vi "ResistanceEquivalent.vi"(3 "Connect":enum16{"SZEREGOWO", "RÓWNOLEGLE"}(ring) caption="Rodzaj po³¹czenia", 4 "R":dbl[](array[numeric]) caption="R [Ohm]") -> (0 "R_eq":dbl caption="R_Z [Ohm]" format="%#.2g")   [LabVIEW 2020]
doc: "Ten subVI liczy opór zastepczy."
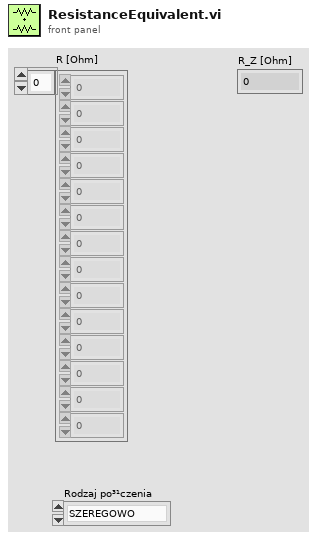
[diagram p1: front panel]
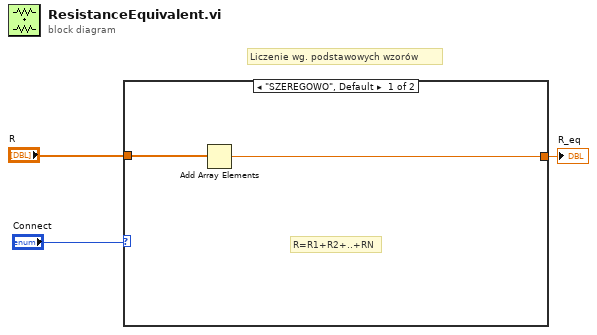
[diagram p0: block diagram]
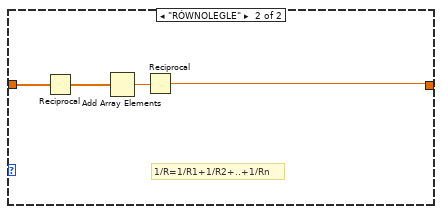
[diagram p2: hidden frame]
diagram:
  # "Liczenie wg. podstawowych wzorów"
  n1 = case shown="\"SZEREGOWO\", Default" "Connect" {
    tunnel: "R" -> [w5 w9]
    tunnel: [w4 w6] -> w1
    frame "SZEREGOWO", Default {
      # "R=R1+R2+..+RN"
      n2 = Add Array Elements(numeric array=w5) -> (sum=w4:dbl)
    }
    frame "RÓWNOLEGLE" {
      # "1/R=1/R1+1/R2+..+1/Rn"
      n3 = Reciprocal(x=w9) -> (1/x=w8:dbl[])
      n4 = Add Array Elements(numeric array=w8) -> (sum=w7:dbl)
      n5 = Reciprocal(x=w7) -> (1/x=w6:dbl)
    }
  }
  "R_eq" <- w1
